vi "Standard Type String To Enum.vi"(1 "Standard Type":T1) -> (0 "Standard Type":T2)   [LabVIEW 2023, in "ACM 4509 Cal Standard.lvlib" / "Cal Standard.lvclass"]
uses:
  Cal Standard.lvclass
  Instruments/Cal Standard/Type Definitions/Standard Type.ctl
  Dependencies/ACM/API/Controls/ACM S-Parameters.ctl
  Instruments/RFFixtureCharact.Instruments.lvlib
  Dependencies/ACM/ACM Visa Driver.lvlib
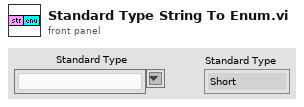
[diagram p1: front panel]
types:
  T1 = typedef "ACM Visa Driver.lvlib/ACM S-Parameters.ctl" = string
  T2 = typedef "RFFixtureCharact.Instruments.lvlib/Standard Type.ctl" = enum16{"Short", "Open", "Load"}
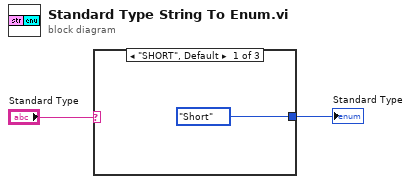
[diagram p0: block diagram]
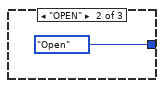
[diagram p2: hidden frame]
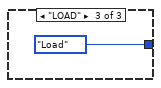
[diagram p3: hidden frame]
diagram:
  n1 = case shown="\"SHORT\", Default" "Standard Type" {
    tunnel: [Standard_Type."Short" ("Standard Type") Standard_Type."Open" ("Standard Type") Standard_Type."Load" ("Standard Type")] -> w1
    frame "SHORT", Default {
    }
    frame "OPEN" {
    }
    frame "LOAD" {
    }
  }
  "Standard Type" <- w1
